vi "e.gate Initialize.vi"(6 "Buffer Index":i32, 7 "eGateHighspeedPortDLLDLL Path":path, 8 "error in (no error)":errorcluster, 10 "Protocol":T5, 11 "IP Address":string) -> (0 "error out":errorcluster, 3 "e.gate Configuration":T2)   [LabVIEW 2016]
doc: "<B>Gantner Instruments Test and Measurement GmbH</B>\n\nLabVIEW Driver for Gantner Instruments e.series controller\n\nThis VI initializes and opens the TCP/IP interface specified by <B>IP address</B>.\n\nIt can be used for ASCII TCP/IP and HighspeedPort TCP/IP which has to be defined with <B>Protocol</B>\nThe name of every VI indicates the protocol it can be used for.\nSome VI's are usable for every protocol and will detect it autimatically.\n\n<B>Buffer Index</B> defines the Buffer"
uses:
  e.gate Protocol Type.ctl
  e.gate Configuration.ctl
  e.gate Channel Data.ctl
  e.gate Data Type.ctl
  e.gate Module  Data.ctl
  e.gateHSP_DLLhandle.ctl
panel:
  in  "DataSource":T1(ring)
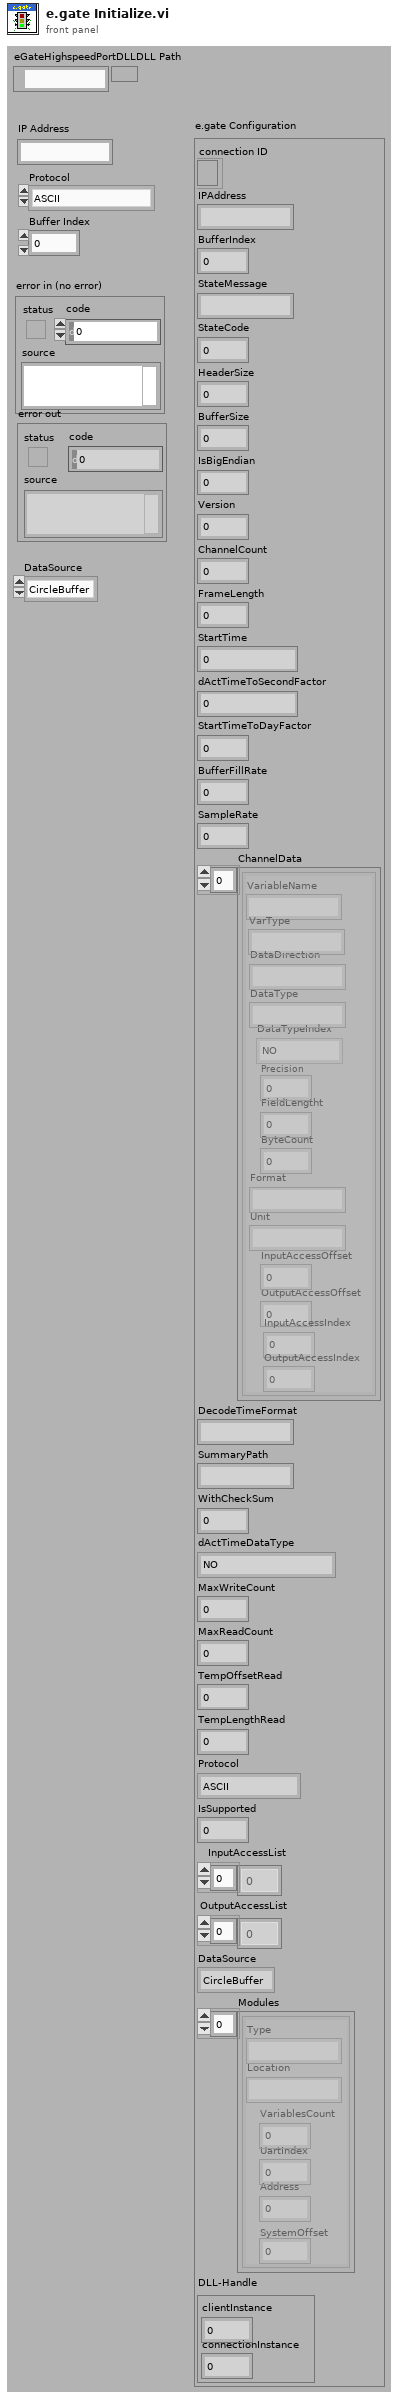
[diagram p1: front panel]
types:
  T1 = enum16{"CircleBuffer", "test.con Logger", "test.con Archive"}
  T2 = typedef "e.gate Configuration.ctl" = cluster{"connection ID":refnum<k5>, "IPAddress":string, "BufferIndex":i32, "StateMessage":string, "StateCode":i8, "HeaderSize":i32, "BufferSize":i32, "IsBigEndian":i32, "Version":i32, "ChannelCount":i32, "FrameLength":i32, "StartTime":dbl, "dActTimeToSecondFactor":dbl, "StartTimeToDayFactor":dbl, "BufferFillRate":dbl, "SampleRate":dbl, "ChannelData":T3[], "DecodeTimeFormat":string, "SummaryPath":string, "WithCheckSum":i32, "dActTimeDataType":T4, "MaxWriteCount":i32, "MaxReadCount":i32, "TempOffsetRead":i32, "TempLengthRead":i32, "Protocol":T5, "IsSupported":i32, "InputAccessList":i32[], "OutputAccessList":i32[], "DataSource":enum16{"CircleBuffer", "test.con Logger", "test.con Archive"}, "Modules":T6[], "DLL-Handle":T7}
  T3 = typedef "e.gate Channel Data.ctl" = cluster{"VariableName":string, "DataDirection":string, "DataType":string, "DataTypeIndex":T4, "Precision":i16, "FieldLengtht":i16, "ByteCount":i32, "Format":string, "Unit":string, "InputAccessOffset":i32, "OutputAccessOffset":i16, "InputAccessIndex":i16, "OutputAccessIndex":i16, "VarType":string}
  T4 = typedef "e.gate Data Type.ctl" = enum16{"NO", "BOOL", "SINT8", "USINT8", "SINT16", "USINT16", "SINT32", "USINT32", "FLOAT", "SET8", "SET16", "SET32", "DOUBLE", "SINT64", "USINT64", "SET64"}
  T5 = typedef "e.gate Protocol Type.ctl" = enum16{"ASCII", "HighspeedPort Online", "HighspeedPort Buffer", "eGateHighspeedPortDLL "}
  T6 = typedef "e.gate Module  Data.ctl" = cluster{"Type":string, "Location":string, "VariablesCount":i16, "UartIndex":i16, "Address":i16, "SystemOffset":i16}
  T7 = typedef "e.gateHSP_DLLhandle.ctl" = cluster{"clientInstance":i32, "connectionInstance":i32}
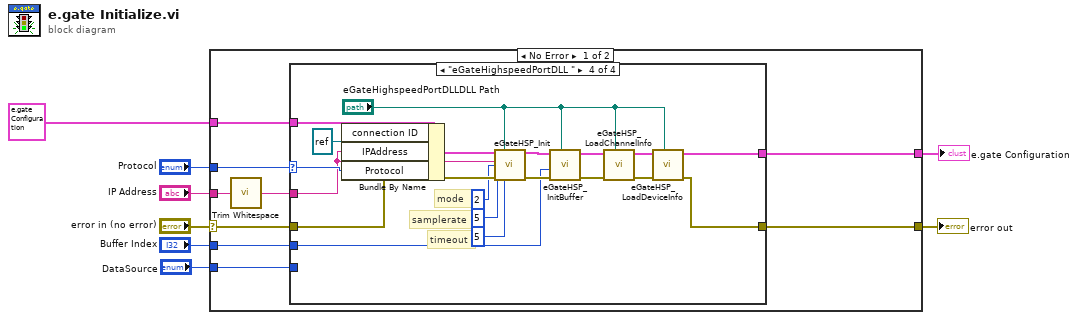
[diagram p0: block diagram]
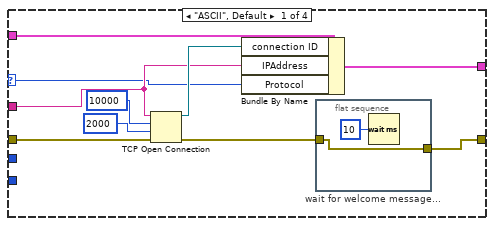
[diagram p2: hidden frame]
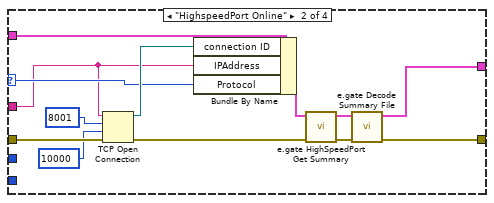
[diagram p3: hidden frame]
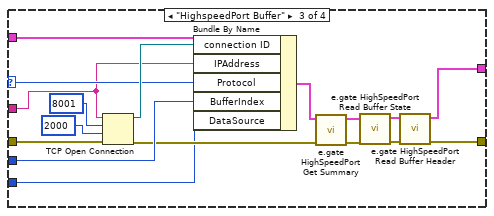
[diagram p4: hidden frame]
diagram:
  n1 = case shown="No Error" "error in (no error)" {
    selector: "error in (no error)" -> [w17 w79]
    tunnel: "IP Address" -> [w12 _]
    tunnel: [w9 w79] -> w6
    tunnel: "Protocol" -> [w16 _]
    tunnel: T2 {"connection ID"=refnum, "IPAddress"="", "BufferIndex"=0, "StateMessage"="", "StateCode"=0, "HeaderSize"=0, "BufferSize"=0, "IsBigEndian"=0, "Version"=0, "ChannelCount"=0, "FrameLength"=0, "StartTime"=0.0, "dActTimeToSecondFactor"=0.0, "StartTimeToDayFactor"=0.0, "BufferFillRate"=0.0, "SampleRate"=0.0, "ChannelData"=[], "DecodeTimeFormat"="", "SummaryPath"="", "WithCheckSum"=0, "dActTimeDataType"=enum."NO", "MaxWriteCount"=0, "MaxReadCount"=0, "TempOffsetRead"=0, "TempLengthRead"=0, "Protocol"=enum."ASCII", "IsSupported"=0, "InputAccessList"=[], "OutputAccessList"=[], "DataSource"=enum."CircleBuffer", "Modules"=[], "DLL-Handle"={"clientInstance"=0, "connectionInstance"=0}} ("e.gate Configuration") -> [w15 _]
    tunnel: [w14 _] -> w3
    tunnel: "Buffer Index" -> [w13 _]
    tunnel: "DataSource" -> [w10 _]
    frame No Error {
      n2 = call <vilib>:"Trim Whitespace.vi"("string"=w12) -> ("trimmed string"=w11:string)  [unwired: 1 in]
      n3 = case shown="\"eGateHighspeedPortDLL \"" w16 {
        selector: w16 -> [w22 w38 w55 w78]
        tunnel: w11 -> [w23 w31 w45 w70]
        tunnel: w17 -> [w26 w41 w58 w74]
        tunnel: [w19 w34 w53 w61] -> w9
        tunnel: w15 -> [w25 w40 w57 w77]
        tunnel: [w21 w32 w51 w62] -> w14
        tunnel: w13 -> [_ _ w50 w67]
        tunnel: w10 -> [_ _ w44 _]
        frame "ASCII", Default {
          n4 = TCP Open Connection(address=w23, remote port or service name=u16 10000, timeout ms (60000)=2000 ("Timeout in ms (60000)"), error in (no error)=w26) -> (connection ID=w24:refnum<k5>, error out=w20:errorcluster)  [unwired: 1 out]
          n5 = Bundle By Name(cluster=w25, "connection ID"=w24, "IPAddress"=w23, "Protocol"=w22) -> (w21:T2)
          n6 = flat-sequence "wait for welcome message..." {
            tunnel: [w28] -> w19
            tunnel: w20 -> [w28]
            frame #0 {
              n7 = Wait (ms)(milliseconds to wait=u32 10) -> ()  [unwired: 1 out]
            }
          }
        }
        frame "HighspeedPort Online" {
          n8 = TCP Open Connection(address=w31, remote port or service name=u16 8001, timeout ms (60000)=10000 ("Timeout in ms (60000)"), error in (no error)=w41) -> (connection ID=w39:refnum<k5>, error out=w37:errorcluster)  [unwired: 1 out]
          n9 = Bundle By Name(cluster=w40, "connection ID"=w39, "IPAddress"=w31, "Protocol"=w38) -> (w36:T2)
          n10 = call "e.gate HighSpeedPort Get Summary.vi"("error in (no error)"=w37, "Configuration in"=w36) -> ("error out"=w35:errorcluster, "Configuration out"=w33:T2)  [unwired: 1 in, 7 out]
          n11 = call "e.gate Decode Summary File.vi"("error in (no error)"=w35, "e.gate Configuration In"=w33) -> ("error out"=w34:errorcluster, "e.gate Configuration Out"=w32:T2)  [unwired: 8 out]
        }
        frame "HighspeedPort Buffer" {
          n12 = TCP Open Connection(address=w45, remote port or service name=u16 8001, timeout ms (60000)=2000 ("Timeout in ms (60000)"), error in (no error)=w58) -> (connection ID=w56:refnum<k5>, error out=w48:errorcluster)  [unwired: 1 out]
          n13 = Bundle By Name(cluster=w57, "connection ID"=w56, "IPAddress"=w45, "Protocol"=w55, "BufferIndex"=w50, "DataSource"=w44) -> (w46:T2)
          n14 = call "e.gate HighSpeedPort Get Summary.vi"("error in (no error)"=w48, "Configuration in"=w46) -> ("error out"=w49:errorcluster, "Configuration out"=w47:T2)  [unwired: 1 in, 7 out]
          n15 = call "e.gate HighSpeedPort Read Buffer State.vi"("error in (no error)"=w49, "Configuration in"=w47) -> ("Error out"=w54:errorcluster, "Configuration out"=w52:T2)  [unwired: 8 out]
          n16 = call "e.gate HighSpeedPort Read Buffer Header.vi"("error in (no error)"=w54, "Configuration in"=w52) -> ("error out"=w53:errorcluster, "Configuration out"=w51:T2)  [unwired: 8 out]
        }
        frame "eGateHighspeedPortDLL " {
          # "mode"
          # "samplerate"
          # "timeout"
          n17 = Bundle By Name(cluster=w77, "connection ID"=refnum<k5> refnum, "IPAddress"=w70, "Protocol"=w78) -> (w75:T2)
          n18 = call "eGateHSP_Init.vi"("e.gate Configuration"=w75, "DLL Path"="eGateHighspeedPortDLLDLL Path", "IP-Adresse"=w70, "mode"=2, "sampleRate"=5, "error in"=w74, "timeout"=5) -> ("e.gate Configuration 2"=w68:T2, "Fehler (Ausgang)"=w69:errorcluster)  [unwired: 7 in]
          n19 = call "eGateHSP_InitBuffer.vi"("path in"="eGateHighspeedPortDLLDLL Path", "Fehler (Eingang, kein Fehler)"=w69, "bufferIndex"=w67, "e.gate Configuration"=w68) -> ("Fehler (Ausgang)"=w66:errorcluster, "e.gate Configuration 2"=w65:T2)  [unwired: 6 in]
          n20 = call "eGateHSP_LoadChannelInfo.vi"("path in"="eGateHighspeedPortDLLDLL Path", "Fehler (Eingang, kein Fehler)"=w66, "e.gate Configuration"=w65) -> ("Fehler (Ausgang)"=w64:errorcluster, "e.gate Configuration 2"=w63:T2)  [unwired: 7 in]
          n21 = call "eGateHSP_LoadDeviceInfo.vi"("path in"="eGateHighspeedPortDLLDLL Path", "Fehler (Eingang, kein Fehler)"=w64, "e.gate Configuration"=w63) -> ("Fehler (Ausgang)"=w61:errorcluster, "e.gate Configuration 2"=w62:T2)  [unwired: 7 in]
        }
      }
    }
    frame Error {
    }
  }
  "error out" <- w6
  "e.gate Configuration" <- w3
